vi "Event Last Ack.vi"(10 "Event Actor":refnum<class "Event Actor.lvclass">, 11 "jettl Queue Actor in":refnum<class "jettl Queue Actor.lvclass">) -> (3 "jettl Queue Actor out":refnum<class "jettl Queue Actor.lvclass">)   [LabVIEW 2021, in "jettl.lvlib" / "jettl Queue Actor.lvclass"]
uses:
  jettl Queue Actor.lvclass
  Actor/Event Actor/Event Actor.lvclass
  jettl Queue Actor.lvclass/jettl Queue Actor.ctl
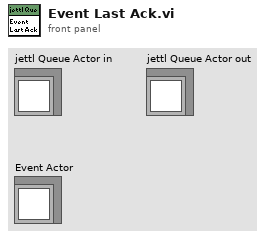
[diagram p1: front panel]
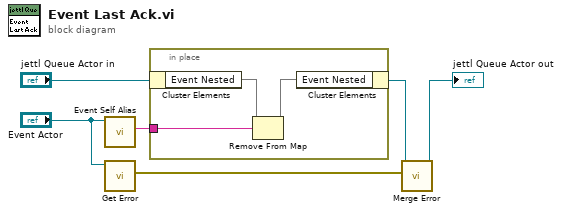
[diagram p0: block diagram]
diagram:
  n1 = call-dynamic "Event Self Alias.vi"("Actor in"="Event Actor") -> ("Event Self Alias"=w1:string)  [unwired: 10 in]
  n2 = call-dynamic "Get Error.vi"("Actor in"="Event Actor") -> ("Error"=w6:errorcluster)  [unwired: 10 in]
  n3 = in-place {
    in-place-border: w1 -> [w7]
    n4 = in-place-cluster #1("jettl Queue Actor in") -> ("Event Nested"=w8:map{string, refnum<data-value>})
    n5 = Remove From Map(10:w7, 11:w8) -> (3:w9:map{string, refnum<data-value>})  [unwired: 2 out]
    n6 = in-place-cluster #1("Event Nested"=w9) -> (w5:refnum<class "jettl Queue Actor.lvclass">)
  }
  n7 = call-dynamic "Merge Error.vi"("Error"=w6, "jettl Queue Actor in"=w5) -> ("jettl Queue Actor out"=→"jettl Queue Actor out":refnum<class "jettl Queue Actor.lvclass">)  [unwired: 9 in]
